vi "Periodic Tasks.vi"(8 "error in":errorcluster) -> ()   [LabVIEW 2020]
doc: "This VI runs in parallel to other tasks. It can contain as many user-defined periodic loops as you need. These can carry out PID or other sorts of timed response."
uses:
  2017 Swerve Code/Swerve Global Variables.vi
  Robot Global Data.vi
  <vilib>/Rock Robotics/WPI/ThirdParty/Sensors/navX/_Processing Loop/FRIC_navX_Internal_SPI_ProcessingLoop.vi
  <vilib>/Rock Robotics/WPI/Solenoid/WPI_SolenoidSetEnum.vi
  <vilib>/Rock Robotics/WPI/Solenoid/WPI_SolenoidValue.ctl
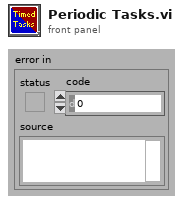
[diagram p1: front panel]
types:
  T1 = typedef "WPI_MotorControlDeviceRef.ctl" = cluster{"DeviceStatus":errorcluster, "Type":T2, "PWM":cluster{"PWM Channel":T3, "DeadBand":T4}, "CAN":cluster{"Device Number":u8, "SetOutput VI Ref":variant, "GetOutput VI Ref":variant, "Enable VI Ref":variant, "Disable VI Ref":variant, "Data":variant}, "Invert":bool, "DIO PWM":cluster{"PWM \"Enable\" Channel":T3, "DIOChannel":T5, "PWM Rate":dbl}}
  T2 = typedef "WPI_MotorControlType.ctl" = enum16{"PWM", "CAN", "DIO PWM"}
  T3 = typedef "FPGA_DIOPWMChannel.ctl" = enum8{"PWM 0", "PWM 1", "PWM 2", "PWM 3", "PWM 4", "PWM 5", "PWM 6", "PWM 7", "PWM 8", "PWM 9", "PWM MXP 0", "PWM MXP 1", "PWM MXP 2", "PWM MXP 3", "PWM MXP 4", "PWM MXP 5", "PWM MXP 6", "PWM MXP 7", "PWM MXP 8", "PWM MXP 9", "Invalid"}
  T4 = typedef "WPI_PWMDeadband.ctl" = cluster{"Name":string, "maxPositivePwm":i32, "minPositivePwm":i32, "centerPwm":i32, "maxNegativePwm":i32, "minNegativePwm":i32, "angularRange":u16}
  T5 = typedef "FPGA_DIOChannel.ctl" = enum8{"DIO 0", "DIO 1", "DIO 2", "DIO 3", "DIO 4", "DIO 5", "DIO 6", "DIO 7", "DIO 8", "DIO 9", "DIO MXP 0", "DIO MXP 1", "DIO MXP 2", "DIO MXP 3", "DIO MXP 4", "DIO MXP 5", "DIO MXP 6", "DIO MXP 7", "DIO MXP 8", "DIO MXP 9", "DIO MXP 10", "DIO MXP 11", "DIO MXP 12", "DIO MXP 13", "DIO MXP 14", "DIO MXP 15", "SPI Port CS1", "SPI Port CS2", "SPI Port CS3", "SPI Port MISO", "SPI Port MOSI", "Invalid"}
  T6 = typedef "WPI_SolenoidDevRef.ctl" = cluster{"DevStatus":errorcluster, "Pneumatics Control Module":u8, "Forward Solenoid Channel":T7, "Reverse Solenoid Channel":T7}
  T7 = typedef "WPI_SolenoidChannel.ctl" = enum8{"Solenoid 0", "Solenoid 1", "Solenoid 2", "Solenoid 3", "Solenoid 4", "Solenoid 5", "Solenoid 6", "Solenoid 7", "Solenoid 8", "Solenoid 9", "Solenoid 10", "Solenoid 11", "Solenoid 12", "Solenoid 13", "Solenoid 14", "Solenoid 15", "Invalid"}
  T8 = typedef "WPI_EncoderDevRef.ctl" = cluster{"DevStatus":errorcluster, "EncoderIndex":T9, "CounterIndex":T10, "DistancePerCount":dbl, "Decoding Type":T11}
  T9 = typedef "FPGA_EncoderIdx.ctl" = enum8{"Enc 0", "Enc 1", "Enc 2", "Enc 3", "Enc 4", "Enc 5", "Enc 6", "Enc 7", "Invalid"}
  T10 = typedef "FPGA_CounterCtrSystemIndex.ctl" = enum8{"Ctr 0", "Ctr 1", "Ctr 2", "Ctr 3", "Ctr 4", "Ctr 5", "Ctr 6", "Ctr 7", "Invalid"}
  T11 = typedef "WPI_EncoderType.ctl" = enum16{"1x", "2x", "4x"}
  T12 = typedef "WPI_CounterDevRef.ctl" = cluster{"DevStatus":errorcluster, "CntIndex":T10}
  T13 = typedef "WPI_SwitchDevRef.ctl" = cluster{"DevStatus":errorcluster, "DIO Channel":T5, "CntIndex":T10, "Normally Closed":bool}
  T14 = typedef "WPI_SolenoidValue.ctl" = enum16{"Off", "On", "Forward", "Reverse"}
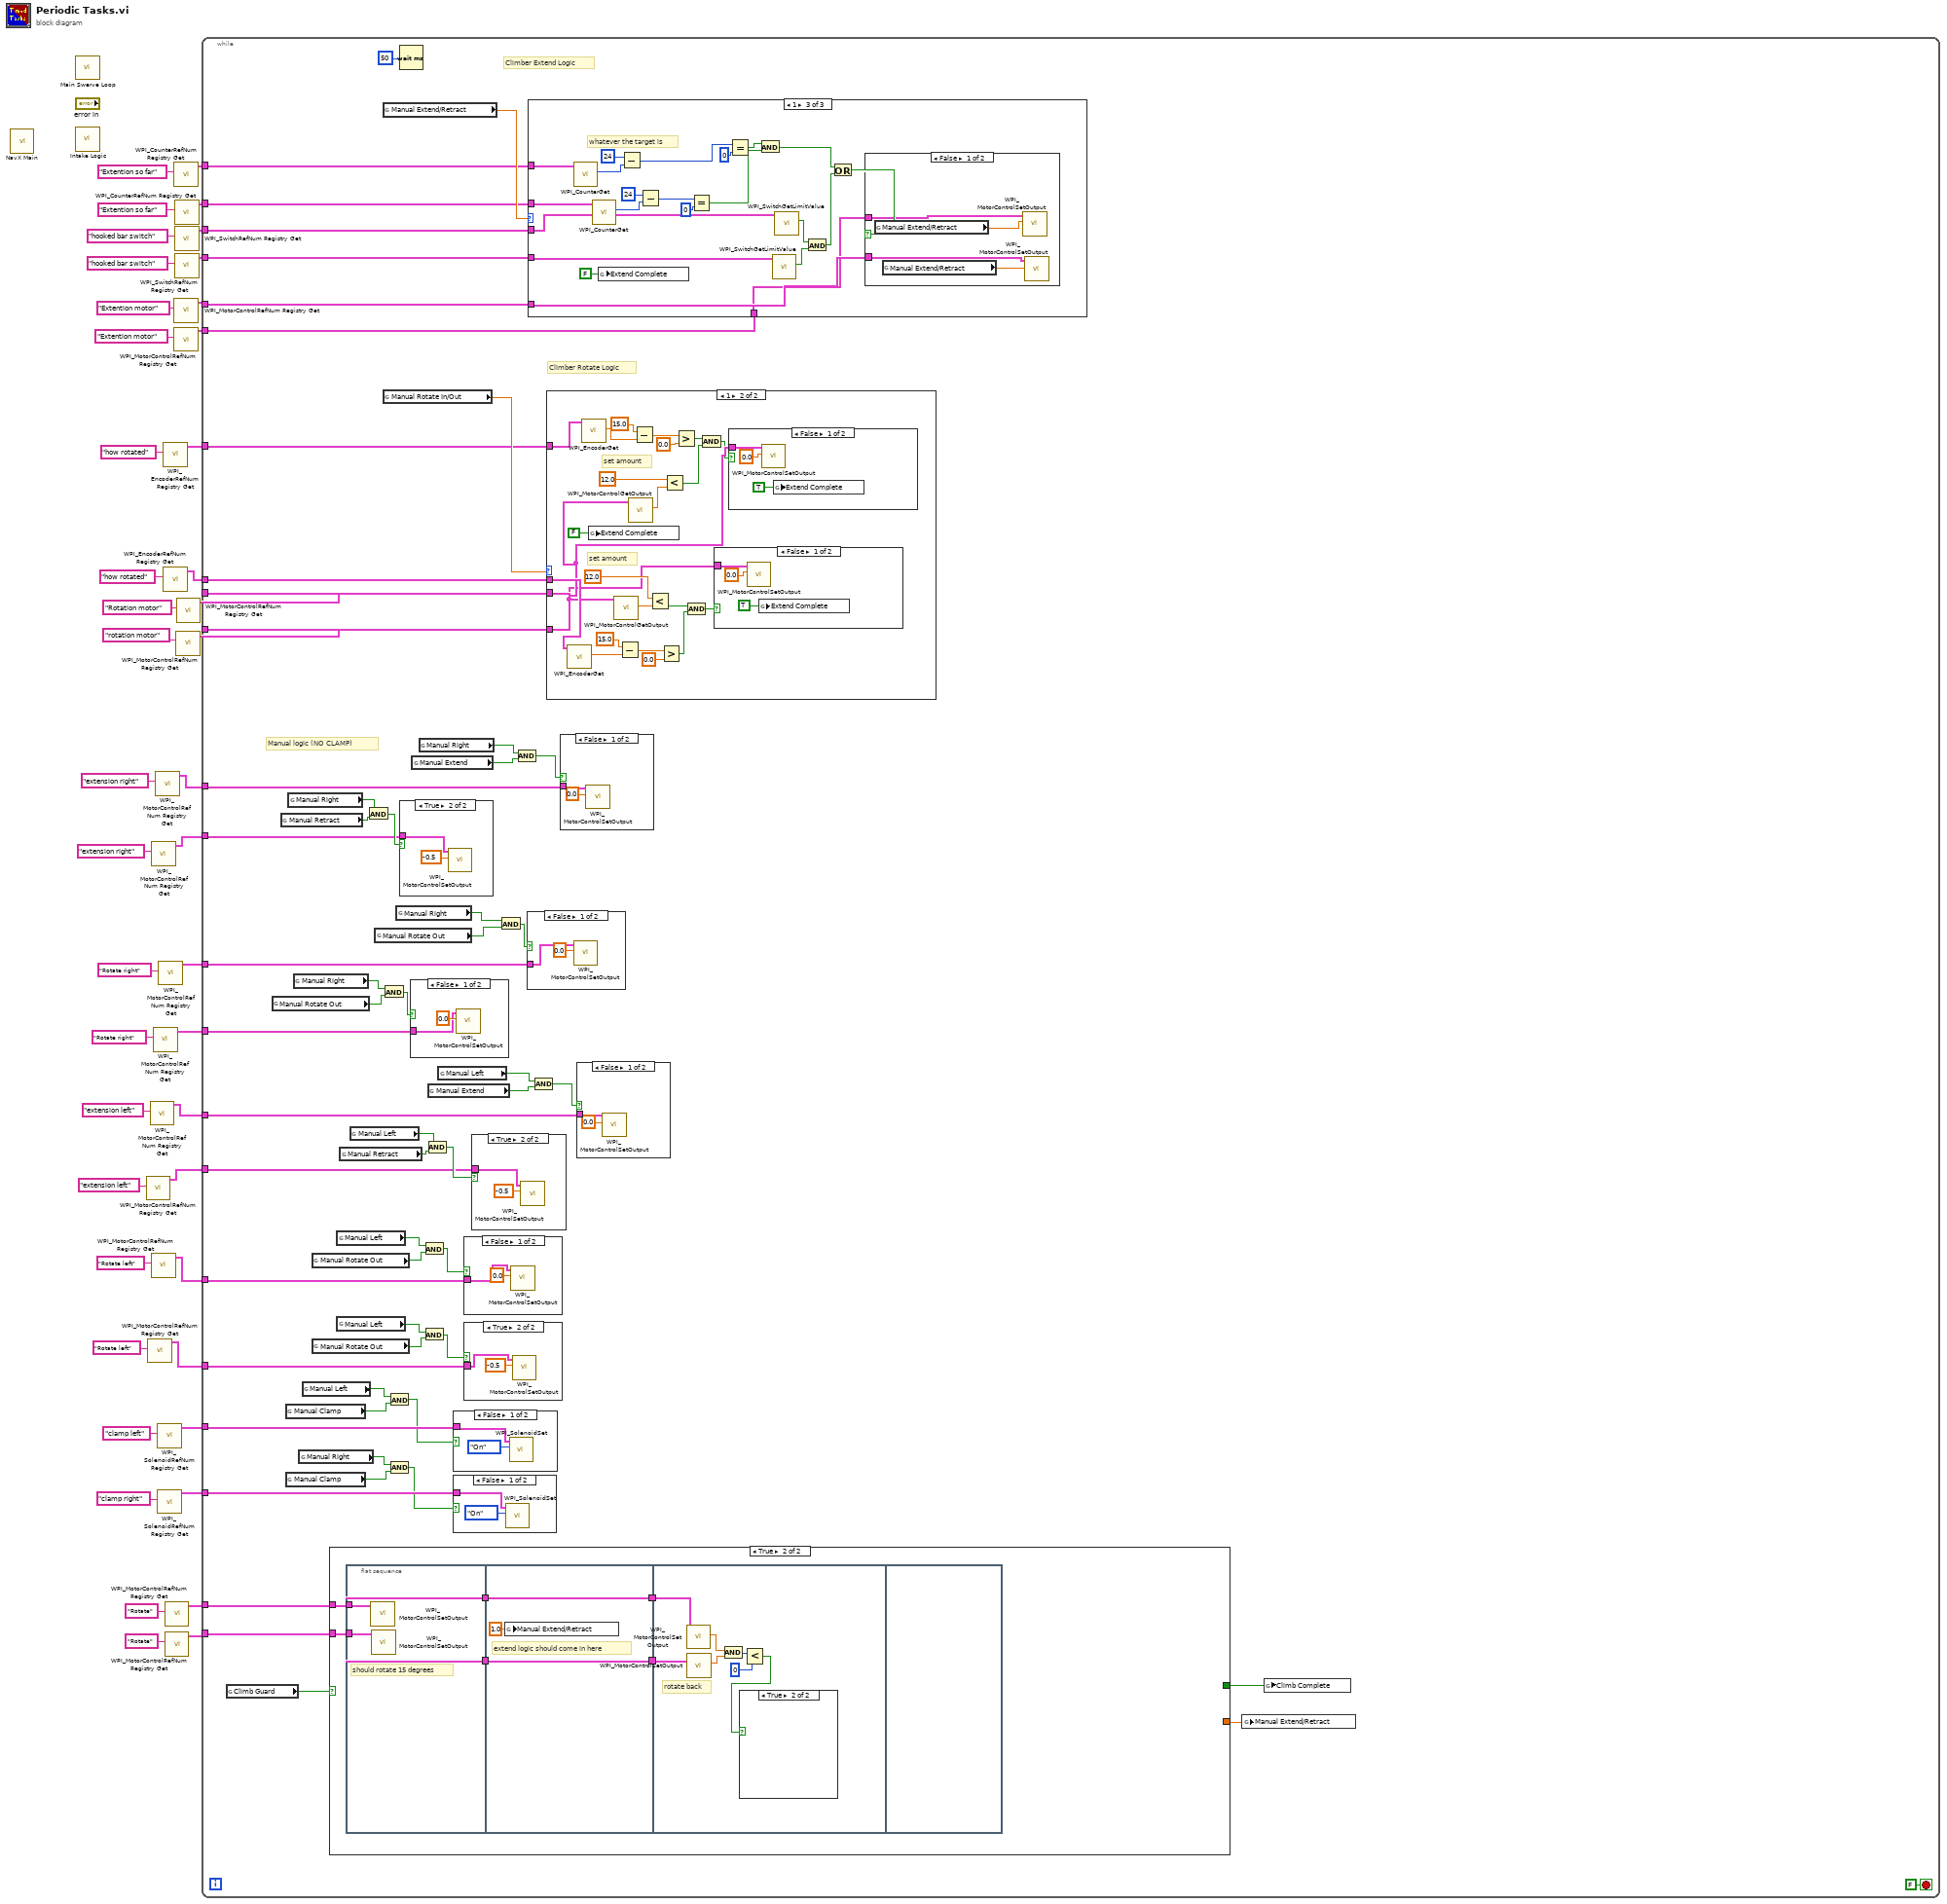
[diagram p0: block diagram]
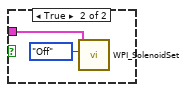
[diagram p2: hidden frame]
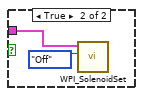
[diagram p3: hidden frame]
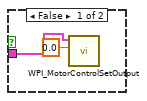
[diagram p4: hidden frame]
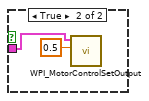
[diagram p5: hidden frame]
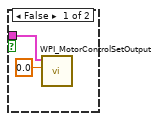
[diagram p6: hidden frame]
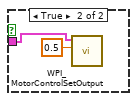
[diagram p7: hidden frame]
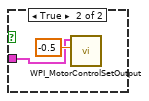
[diagram p8: hidden frame]
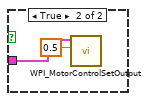
[diagram p9: hidden frame]
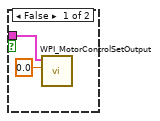
[diagram p10: hidden frame]
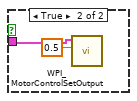
[diagram p11: hidden frame]
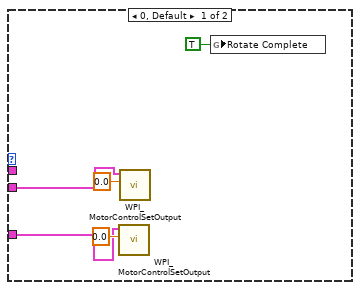
[diagram p12: hidden frame]
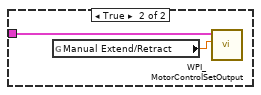
[diagram p13: hidden frame]
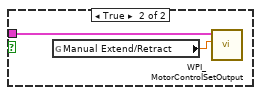
[diagram p14: hidden frame]
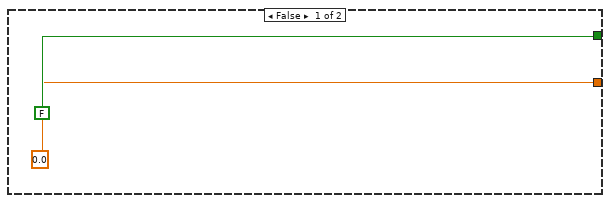
[diagram p15: hidden frame]
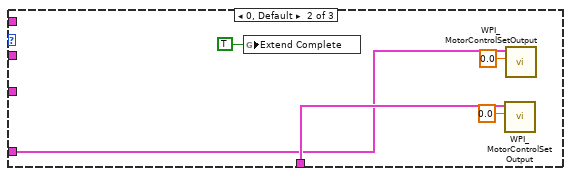
[diagram p18: hidden frame]
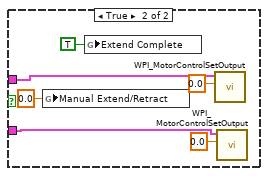
[diagram p19: hidden frame]
diagram:
  n1 = call-poly <vilib>:"NavX Main.vi"() -> ()  [unwired: 12 in]
  n2 = call "Main Swerve Loop.vi"() -> ()  [unwired: 12 in]
  n3 = call "Intake Logic.vi"() -> ()  [unwired: 12 in]
  n4 = call <vilib>:"WPI_MotorControlRefNum Registry Get.vi"("refnum name"="extension left") -> ("MotorControlDevRef"=w7:T1)  [unwired: 9 in, 1 out]
  n5 = call <vilib>:"WPI_MotorControlRefNum Registry Get.vi"("refnum name"="Rotate left") -> ("MotorControlDevRef"=w5:T1)  [unwired: 9 in, 1 out]
  n6 = call <vilib>:"WPI_MotorControlRefNum Registry Get.vi"("refnum name"="extension left") -> ("MotorControlDevRef"=w8:T1)  [unwired: 9 in, 1 out]
  n7 = call <vilib>:"WPI_MotorControlRefNum Registry Get.vi"("refnum name"="extension right") -> ("MotorControlDevRef"=w13:T1)  [unwired: 9 in, 1 out]
  n8 = call <vilib>:"WPI_MotorControlRefNum Registry Get.vi"("refnum name"="Rotate left") -> ("MotorControlDevRef"=w6:T1)  [unwired: 9 in, 1 out]
  n9 = call <vilib>:"WPI_MotorControlRefNum Registry Get.vi"("refnum name"="Rotate right") -> ("MotorControlDevRef"=w15:T1)  [unwired: 9 in, 1 out]
  n10 = call <vilib>:"WPI_MotorControlRefNum Registry Get.vi"("refnum name"="extension right") -> ("MotorControlDevRef"=w19:T1)  [unwired: 9 in, 1 out]
  n11 = call <vilib>:"WPI_SolenoidRefNum Registry Get.vi"("refnum name"="clamp left") -> ("SolenoidDevRef"=w4:T6)  [unwired: 9 in, 1 out]
  n12 = call <vilib>:"WPI_SolenoidRefNum Registry Get.vi"("refnum name"="clamp right") -> ("SolenoidDevRef"=w3:T6)  [unwired: 9 in, 1 out]
  n13 = call <vilib>:"WPI_MotorControlRefNum Registry Get.vi"("refnum name"="Rotate right") -> ("MotorControlDevRef"=w17:T1)  [unwired: 9 in, 1 out]
  n14 = call <vilib>:"WPI_EncoderRefNum Registry Get.vi"("refnum name"="how rotated") -> ("EncoderDevRef"=w28:T8)  [unwired: 9 in, 1 out]
  n15 = call <vilib>:"WPI_EncoderRefNum Registry Get.vi"("refnum name"="how rotated") -> ("EncoderDevRef"=w27:T8)  [unwired: 9 in, 1 out]
  n16 = call <vilib>:"WPI_MotorControlRefNum Registry Get.vi"("refnum name"="Rotate") -> ("MotorControlDevRef"=w44:T1)  [unwired: 9 in, 1 out]
  n17 = call <vilib>:"WPI_MotorControlRefNum Registry Get.vi"("refnum name"="Rotate") -> ("MotorControlDevRef"=w41:T1)  [unwired: 9 in, 1 out]
  n18 = call <vilib>:"WPI_CounterRefNum Registry Get.vi"("refnum name"="Extention so far") -> ("CounterDevRef"=w40:T12)  [unwired: 9 in, 1 out]
  n19 = call <vilib>:"WPI_MotorControlRefNum Registry Get.vi"("refnum name"="Extention motor") -> ("MotorControlDevRef"=w38:T1)  [unwired: 9 in, 1 out]
  n20 = call <vilib>:"WPI_MotorControlRefNum Registry Get.vi"("refnum name"="Extention motor") -> ("MotorControlDevRef"=w37:T1)  [unwired: 9 in, 1 out]
  n21 = call <vilib>:"WPI_CounterRefNum Registry Get.vi"("refnum name"="Extention so far") -> ("CounterDevRef"=w39:T12)  [unwired: 9 in, 1 out]
  n22 = call <vilib>:"WPI_SwitchRefNum Registry Get.vi"("refnum name"="hooked bar switch") -> ("SwitchDevRef"=w30:T13)  [unwired: 9 in, 1 out]
  n23 = call <vilib>:"WPI_SwitchRefNum Registry Get.vi"("refnum name"="hooked bar switch") -> ("SwitchDevRef"=w29:T13)  [unwired: 9 in, 1 out]
  n24 = call <vilib>:"WPI_MotorControlRefNum Registry Get.vi"("refnum name"="rotation motor") -> ("MotorControlDevRef"=w21:T1)  [unwired: 9 in, 1 out]
  n25 = call <vilib>:"WPI_MotorControlRefNum Registry Get.vi"("refnum name"="Rotation motor") -> ("MotorControlDevRef"=w22:T1)  [unwired: 9 in, 1 out]
  n26 = while {
    tunnel: w44 -> [w97]
    tunnel: w41 -> [w96]
    tunnel: w40 -> [w95]
    tunnel: w39 -> [w94]
    tunnel: w38 -> [w93]
    tunnel: w37 -> [w92]
    tunnel: w30 -> [w91]
    tunnel: w29 -> [w90]
    tunnel: w28 -> [w88]
    tunnel: w27 -> [w87]
    tunnel: w22 -> [w86]
    tunnel: w21 -> [w85]
    tunnel: w19 -> [w81]
    tunnel: w17 -> [w74]
    tunnel: w15 -> [w70]
    tunnel: w13 -> [w69]
    tunnel: w8 -> [w56]
    tunnel: w7 -> [w55]
    tunnel: w6 -> [w54]
    tunnel: w5 -> [w53]
    tunnel: w4 -> [w52]
    tunnel: w3 -> [w51]
    stop <- FALSE stop-if-true
    # "Manual logic (NO CLAMP)"
    # "Climber Rotate Logic"
    # "Climber Extend Logic"
    n27 = global read "Robot Global Data.vi" "Climb Guard"() -> (w100:bool)
    n28 = global read "Robot Global Data.vi" "Manual Rotate Out"() -> (w71:bool)
    n29 = global read "Robot Global Data.vi" "Manual Retract"() -> (w79:bool)
    n30 = global read "Robot Global Data.vi" "Manual Clamp"() -> (w49:bool)
    n31 = global read "Robot Global Data.vi" "Manual Clamp"() -> (w47:bool)
    n32 = global read "Robot Global Data.vi" "Manual Right"() -> (w80:bool)
    n33 = global read "Robot Global Data.vi" "Manual Right"() -> (w72:bool)
    n34 = global read "Robot Global Data.vi" "Manual Right"() -> (w48:bool)
    n35 = global read "Robot Global Data.vi" "Manual Left"() -> (w50:bool)
    n36 = global read "Robot Global Data.vi" "Manual Rotate Out"() -> (w60:bool)
    n37 = global read "Robot Global Data.vi" "Manual Rotate Out"() -> (w57:bool)
    n38 = case shown="True" w100 {
      tunnel: [FALSE _] -> w99
      tunnel: [0.0 _] -> w98
      tunnel: w97 -> [_ w189]
      tunnel: w96 -> [_ w188]
      frame False {
      }
      frame True {
        n39 = flat-sequence {
          tunnel: w189 -> [w190]
          tunnel: w188 -> [w191]
          tunnel: [w191] -> w186
          tunnel: [w190] -> w184
          tunnel: [w193] -> w187
          tunnel: w186 -> [w193]
          tunnel: [w192] -> w185
          tunnel: w184 -> [w192]
          tunnel: w187 -> [w201]
          tunnel: w185 -> [w200]
          frame #0 {
            # "should rotate 15 degrees"
            n40 = call <vilib>:"WPI_MotorControlSetOutput.vi"("MotorControlDevRef"=w190) -> ()  [unwired: 8 in, 3 out]
            n41 = call <vilib>:"WPI_MotorControlSetOutput.vi"("MotorControlDevRef"=w191) -> ()  [unwired: 8 in, 3 out]
          }
          frame #1 {
            # "extend logic should come in here"
            n42 = global write "Swerve Global Variables.vi" "Manual Extend/Retract"(1.0 ("Manual Extend/Retract")) -> ()
          }
          frame #2 {
            # "rotate back"
            n43 = call <vilib>:"WPI_MotorControlSetOutput.vi"("MotorControlDevRef"=w200) -> ("Motor Output"=w198:dbl)  [unwired: 8 in, 2 out]
            n44 = call <vilib>:"WPI_MotorControlSetOutput.vi"("MotorControlDevRef"=w201) -> ("Motor Output"=w199:dbl)  [unwired: 8 in, 2 out]
            n45 = And(x=w198, y=w199) -> (x .and. y?=w197:i32)
            n46 = Less?(x=w197, y=0) -> (x < y?=w195:bool)
            n47 = case shown="True" w195 {
              frame False {
              }
              frame True {
              }
            }
          }
          frame #3 {
          }
        }
      }
    }
    n48 = global read "Robot Global Data.vi" "Manual Left"() -> (w61:bool)
    n49 = global read "Robot Global Data.vi" "Manual Left"() -> (w58:bool)
    n50 = global read "Robot Global Data.vi" "Manual Retract"() -> (w64:bool)
    n51 = global read "Robot Global Data.vi" "Manual Left"() -> (w65:bool)
    n52 = And(x=w80, y=w79) -> (x .and. y?=w78:bool)
    n53 = global read "Robot Global Data.vi" "Manual Rotate Out"() -> (w75:bool)
    n54 = And(x=w72, y=w71) -> (x .and. y?=w73:bool)
    n55 = global read "Swerve Global Variables.vi" "Manual Extend/Retract"() -> (w101:dbl)
    n56 = global read "Swerve Global Variables.vi" "Manual Rotate In/Out"() -> (w89:dbl)
    n57 = And(x=w50, y=w49) -> (x .and. y?=w45:bool)
    n58 = And(x=w48, y=w47) -> (x .and. y?=w46:bool)
    n59 = global read "Robot Global Data.vi" "Manual Right"() -> (w76:bool)
    n60 = Wait (ms)(milliseconds to wait=u32 50) -> ()  [unwired: 1 out]
    n61 = case shown="True" w78 {
      tunnel: w69 -> [w136 w138]
      frame False {
        n62 = call <vilib>:"WPI_MotorControlSetOutput.vi"("Output"=0.0, "MotorControlDevRef"=w136) -> ()  [unwired: 7 in, 3 out]
      }
      frame True {
        n63 = call <vilib>:"WPI_MotorControlSetOutput.vi"("Output"=-0.5, "MotorControlDevRef"=w138) -> ()  [unwired: 7 in, 3 out]
      }
    }
    n64 = case shown="False" w73 {
      tunnel: w70 -> [w128 w130]
      frame False {
        n65 = call <vilib>:"WPI_MotorControlSetOutput.vi"("Output"=0.0, "MotorControlDevRef"=w128) -> ()  [unwired: 7 in, 3 out]
      }
      frame True {
        n66 = call <vilib>:"WPI_MotorControlSetOutput.vi"("Output"=-0.5, "MotorControlDevRef"=w130) -> ()  [unwired: 7 in, 3 out]
      }
    }
    n67 = global read "Robot Global Data.vi" "Manual Extend"() -> (w84:bool)
    n68 = global read "Robot Global Data.vi" "Manual Right"() -> (w83:bool)
    n69 = And(x=w61, y=w60) -> (x .and. y?=w62:bool)
    n70 = And(x=w58, y=w57) -> (x .and. y?=w59:bool)
    n71 = And(x=w65, y=w64) -> (x .and. y?=w63:bool)
    n72 = global read "Robot Global Data.vi" "Manual Extend"() -> (w68:bool)
    n73 = global read "Robot Global Data.vi" "Manual Left"() -> (w67:bool)
    n74 = case shown="False" w45 {
      tunnel: w52 -> [w108 w111]
      frame False {
        n75 = call-poly <vilib>:"WPI_SolenoidSet.vi"("Value"=WPI_SolenoidValue."On", "SolenoidDevRef"=w108) -> ()  [unwired: 8 in, 2 out]
      }
      frame True {
        n76 = call-poly <vilib>:"WPI_SolenoidSet.vi"("Value"=WPI_SolenoidValue."Off", "SolenoidDevRef"=w111) -> ()  [unwired: 8 in, 2 out]
      }
    }
    n77 = case shown="False" w46 {
      tunnel: w51 -> [w104 w107]
      frame False {
        n78 = call-poly <vilib>:"WPI_SolenoidSet.vi"("Value"=WPI_SolenoidValue."On", "SolenoidDevRef"=w104) -> ()  [unwired: 8 in, 2 out]
      }
      frame True {
        n79 = call-poly <vilib>:"WPI_SolenoidSet.vi"("Value"=WPI_SolenoidValue."Off", "SolenoidDevRef"=w107) -> ()  [unwired: 8 in, 2 out]
      }
    }
    n80 = case shown="False" w62 {
      tunnel: w54 -> [w116 w118]
      frame False {
        n81 = call <vilib>:"WPI_MotorControlSetOutput.vi"("Output"=0.0, "MotorControlDevRef"=w116) -> ()  [unwired: 7 in, 3 out]
      }
      frame True {
        n82 = call <vilib>:"WPI_MotorControlSetOutput.vi"("Output"=0.5, "MotorControlDevRef"=w118) -> ()  [unwired: 7 in, 3 out]
      }
    }
    n83 = case shown="True" w59 {
      tunnel: w53 -> [w112 w114]
      frame False {
        n84 = call <vilib>:"WPI_MotorControlSetOutput.vi"("Output"=0.0, "MotorControlDevRef"=w112) -> ()  [unwired: 7 in, 3 out]
      }
      frame True {
        n85 = call <vilib>:"WPI_MotorControlSetOutput.vi"("Output"=-0.5, "MotorControlDevRef"=w114) -> ()  [unwired: 7 in, 3 out]
      }
    }
    n86 = case shown="True" w63 {
      tunnel: w55 -> [w120 w122]
      frame False {
        n87 = call <vilib>:"WPI_MotorControlSetOutput.vi"("Output"=0.0, "MotorControlDevRef"=w120) -> ()  [unwired: 7 in, 3 out]
      }
      frame True {
        n88 = call <vilib>:"WPI_MotorControlSetOutput.vi"("Output"=-0.5, "MotorControlDevRef"=w122) -> ()  [unwired: 7 in, 3 out]
      }
    }
    n89 = And(x=w76, y=w75) -> (x .and. y?=w77:bool)
    n90 = And(x=w83, y=w84) -> (x .and. y?=w82:bool)
    n91 = case shown="False" w77 {
      tunnel: w74 -> [w133 w135]
      frame False {
        n92 = call <vilib>:"WPI_MotorControlSetOutput.vi"("Output"=0.0, "MotorControlDevRef"=w133) -> ()  [unwired: 7 in, 3 out]
      }
      frame True {
        n93 = call <vilib>:"WPI_MotorControlSetOutput.vi"("Output"=0.5, "MotorControlDevRef"=w135) -> ()  [unwired: 7 in, 3 out]
      }
    }
    n94 = case shown="1" w101 {
      tunnel: w95 -> [_ _ w228]
      tunnel: w94 -> [_ _ w227]
      tunnel: w93 -> [_ w204 w226]
      tunnel: w92 -> [_ w205 w225]
      tunnel: w91 -> [_ _ w224]
      tunnel: w90 -> [_ _ w223]
      frame -1 {
      }
      frame 0, Default {
        n95 = global write "Robot Global Data.vi" "Extend Complete"(TRUE) -> ()
        n96 = call <vilib>:"WPI_MotorControlSetOutput.vi"("Output"=0.0, "MotorControlDevRef"=w205) -> ()  [unwired: 7 in, 3 out]
        n97 = call <vilib>:"WPI_MotorControlSetOutput.vi"("Output"=0.0, "MotorControlDevRef"=w204) -> ()  [unwired: 7 in, 3 out]
      }
      frame 1 {
        # "whatever the target is"
        n98 = call <vilib>:"WPI_CounterGet.vi"("CounterDevRef in"=w228) -> ("Value"=w221:i32)  [unwired: 5 in, 5 out]
        n99 = call <vilib>:"WPI_CounterGet.vi"("CounterDevRef in"=w227) -> ("Value"=w219:i32)  [unwired: 5 in, 5 out]
        n100 = global write "Robot Global Data.vi" "Extend Complete"(FALSE ("Extend Complete")) -> ()
        n101 = Subtract(x=24, y=w221) -> (x-y=w217:i32)
        n102 = Subtract(x=24, y=w219) -> (x-y=w214:i32)
        n103 = Equal?(x=w214, y=0) -> (x = y?=w207:bool)
        n104 = Equal?(x=w217, y=0) -> (x = y?=w213:bool)
        n105 = And(x=w213, y=w207) -> (x .and. y?=w210:bool)
        n106 = call <vilib>:"WPI_SwitchGetLimitValue.vi"("SwitchDevRef"=w223) -> ("Switch Pressed"=w212:bool)  [unwired: 8 in, 2 out]
        n107 = call <vilib>:"WPI_SwitchGetLimitValue.vi"("SwitchDevRef"=w224) -> ("Switch Pressed"=w211:bool)  [unwired: 8 in, 2 out]
        n108 = And(x=w211, y=w212) -> (x .and. y?=w209:bool)
        n109 = Or(x=w210, y=w209) -> (x .or. y?=w208:bool)
        n110 = case shown="False" w208 {
          tunnel: w225 -> [w230 w238]
          tunnel: w226 -> [w229 w237]
          frame False {
            n111 = global read "Swerve Global Variables.vi" "Manual Extend/Retract"() -> (w231:dbl)
            n112 = global read "Swerve Global Variables.vi" "Manual Extend/Retract"() -> (w232:dbl)
            n113 = call <vilib>:"WPI_MotorControlSetOutput.vi"("Output"=w231, "MotorControlDevRef"=w230) -> ()  [unwired: 7 in, 3 out]
            n114 = call <vilib>:"WPI_MotorControlSetOutput.vi"("Output"=w232, "MotorControlDevRef"=w229) -> ()  [unwired: 7 in, 3 out]
          }
          frame True {
            n115 = global write "Swerve Global Variables.vi" "Manual Extend/Retract"(0.0 ("Manual Extend/Retract")) -> ()
            n116 = global write "Robot Global Data.vi" "Extend Complete"(TRUE ("Extend Complete")) -> ()
            n117 = call <vilib>:"WPI_MotorControlSetOutput.vi"("Output"=0.0, "MotorControlDevRef"=w238) -> ()  [unwired: 7 in, 3 out]
            n118 = call <vilib>:"WPI_MotorControlSetOutput.vi"("Output"=0.0, "MotorControlDevRef"=w237) -> ()  [unwired: 7 in, 3 out]
          }
        }
      }
    }
    n119 = And(x=w67, y=w68) -> (x .and. y?=w66:bool)
    n120 = case shown="1" w89 {
      tunnel: w88 -> [_ w171]
      tunnel: w87 -> [_ w170]
      tunnel: w86 -> [w144 w160]
      tunnel: w85 -> [w145 w155]
      frame 0, Default {
        n121 = call <vilib>:"WPI_MotorControlSetOutput.vi"("Output"=0.0, "MotorControlDevRef"=w145) -> ()  [unwired: 7 in, 3 out]
        n122 = call <vilib>:"WPI_MotorControlSetOutput.vi"("Output"=0.0, "MotorControlDevRef"=w144) -> ()  [unwired: 7 in, 3 out]
        n123 = global write "Robot Global Data.vi" "Rotate Complete"(TRUE) -> ()
      }
      frame 1 {
        # "set amount"
        # "set amount"
        n124 = call <vilib>:"WPI_EncoderGet.vi"("EncoderDevRef"=w170) -> ("Distance"=w167:dbl)  [unwired: 5 in, 5 out]
        n125 = call <vilib>:"WPI_EncoderGet.vi"("EncoderDevRef"=w171) -> ("Distance"=w169:dbl)  [unwired: 5 in, 5 out]
        n126 = global write "Robot Global Data.vi" "Extend Complete"(FALSE ("Extend Complete")) -> ()
        n127 = call <vilib>:"WPI_MotorControlGetOutput.vi"("MotorControlDevRef"=w155) -> ("Output"=w157:dbl)  [unwired: 8 in, 2 out]
        n128 = Subtract(x=15.0, y=w167) -> (x-y=w161:dbl)
        n129 = call <vilib>:"WPI_MotorControlGetOutput.vi"("MotorControlDevRef"=w160) -> ("Output"=w159:dbl)  [unwired: 8 in, 2 out]
        n130 = Subtract(x=15.0, y=w169) -> (x-y=w164:dbl)
        n131 = Less?(x=12.0, y=w157) -> (x < y?=w152:bool)
        n132 = Greater?(x=w161, y=0.0) -> (0:w151:bool)
        n133 = Less?(x=12.0, y=w159) -> (x < y?=w154:bool)
        n134 = Greater?(x=w164, y=0.0) -> (0:w153:bool)
        n135 = And(x=w152, y=w151) -> (x .and. y?=w150:bool)
        n136 = And(x=w153, y=w154) -> (x .and. y?=w149:bool)
        n137 = case shown="False" w150 {
          tunnel: w155 -> [w173 w176]
          frame False {
            n138 = call <vilib>:"WPI_MotorControlSetOutput.vi"("Output"=0.0, "MotorControlDevRef"=w173) -> ()  [unwired: 7 in, 3 out]
            n139 = global write "Robot Global Data.vi" "Extend Complete"(TRUE ("Extend Complete")) -> ()
          }
          frame True {
            n140 = global read "Swerve Global Variables.vi" "Manual Extend/Retract"() -> (w175:dbl)
            n141 = call <vilib>:"WPI_MotorControlSetOutput.vi"("Output"=w175, "MotorControlDevRef"=w176) -> ()  [unwired: 7 in, 3 out]
          }
        }
        n142 = case shown="False" w149 {
          tunnel: w160 -> [w179 w181]
          frame False {
            n143 = call <vilib>:"WPI_MotorControlSetOutput.vi"("Output"=0.0, "MotorControlDevRef"=w179) -> ()  [unwired: 7 in, 3 out]
            n144 = global write "Robot Global Data.vi" "Extend Complete"(TRUE ("Extend Complete")) -> ()
          }
          frame True {
            n145 = global read "Swerve Global Variables.vi" "Manual Extend/Retract"() -> (w180:dbl)
            n146 = call <vilib>:"WPI_MotorControlSetOutput.vi"("Output"=w180, "MotorControlDevRef"=w181) -> ()  [unwired: 7 in, 3 out]
          }
        }
      }
    }
    n147 = case shown="False" w82 {
      tunnel: w81 -> [w141 w143]
      frame False {
        n148 = call <vilib>:"WPI_MotorControlSetOutput.vi"("Output"=0.0, "MotorControlDevRef"=w141) -> ()  [unwired: 7 in, 3 out]
      }
      frame True {
        n149 = call <vilib>:"WPI_MotorControlSetOutput.vi"("Output"=0.5, "MotorControlDevRef"=w143) -> ()  [unwired: 7 in, 3 out]
      }
    }
    n150 = case shown="False" w66 {
      tunnel: w56 -> [w124 w126]
      frame False {
        n151 = call <vilib>:"WPI_MotorControlSetOutput.vi"("Output"=0.0, "MotorControlDevRef"=w124) -> ()  [unwired: 7 in, 3 out]
      }
      frame True {
        n152 = call <vilib>:"WPI_MotorControlSetOutput.vi"("Output"=0.5, "MotorControlDevRef"=w126) -> ()  [unwired: 7 in, 3 out]
      }
    }
    n153 = global write "Swerve Global Variables.vi" "Manual Extend/Retract"(w98) -> ()
    n154 = global write "Robot Global Data.vi" "Climb Complete"(w99) -> ()
  }
